vi "PH_SystemInformation.constructor.vi"(0 "name":string, 2 "data in":string, 5 "error in(no error)":errorcluster) -> (14 "i ref out":refnum<vi>, 16 "data out":string, 19 "error out":errorcluster)   [LabVIEW 2014, in "PH_SystemInformation.lvlib"]
doc: "This class is forseen to control black boxes (motion).\n\nThis class is part of the PHELIX device layer.\n\nauthor: Stefan Götte, GSI\n\nLicense Agreement for this software:\n\nCopyright (C)\nGesellschaft für Schwerionenforschung, GSI\nPlanckstr. 1\n64291 Darmstadt\nGermany\n\nContact: D.Beck@gsi.de \n\nThis program is free software; you can redistribute it and/or modify it under the terms of the \nGNU General Public License as published by the Free Software Foundation; either version 2 of \nthe license, or (at your option) any later version.\n\nThis program is distributed in the hope that it will be useful, but WITHOUT ANY WARRANTY; \nwithout even the implied warranty of MERCHANTABILITY or FITNESS FOR A PARTICULAR PURPOSE. See the GNU General License for more details (http://www.gnu.org).\n\nGesellschaft für Schwerionenforschung, GSI\nPlanckstr. 1, 64291 Darmstadt, Germany\nFor all questions and ideas contact: M.Richter@gsi.de, H.Brand@gsi.de or D.Beck@gsi.de.\nLast update: 16-JUN-2004"
uses:
  PH_SystemInformation.lvlib
  CSCore/CSSystem/CSSystemLib/CSSystemLib.lvlib
  PH_Class/PH_Class.lvlib
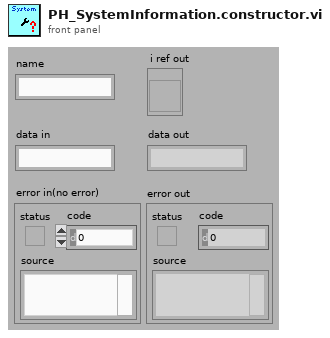
[diagram p1: front panel]
types:
  T1 = enum16{"SetAttribute", "GetAttribute", "CreateAttribute", "DestroyAttribute", "DestroyAllAtributes"}
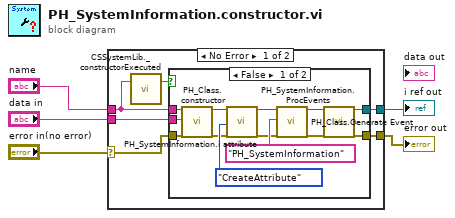
[diagram p0: block diagram]
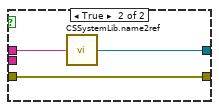
[diagram p2: hidden frame]
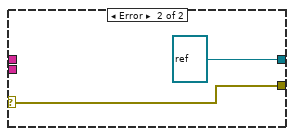
[diagram p3: hidden frame]
diagram:
  n1 = case shown="No Error" "error in(no error)" {
    selector: "error in(no error)" -> [w11 w29]
    tunnel: [w9 refnum<vi> refnum ("i ref out")] -> w5
    tunnel: [w10 w29] -> w4
    tunnel: "name" -> [w8 _]
    tunnel: "data in" -> [w6 _]
    frame No Error {
      n2 = call "CSSystemLib._constructorExecuted.vi"("name"=w8) -> ("constructor executed?"=w7:bool)  [unwired: 18 in]
      n3 = case shown="False" w7 {
        tunnel: w11 -> [w13 w27]
        tunnel: [w23 w27] -> w10
        tunnel: [w22 w25] -> w9
        tunnel: w8 -> [w21 w26]
        tunnel: w6 -> [w12 _]
        frame False {
          n4 = call "PH_Class.constructor.vi"("name"=w21, "data in"=w12, "error in"=w13) -> ("i ref out"=w18:refnum<vi>, "error out"=w19:errorcluster)  [unwired: 14 in, 1 out]
          n5 = call "PH_SystemInformation.i attribute.vi"("VI Refnum"=w18, "Action"=T1."CreateAttribute", "error in (no error)"=w19) -> ("VI Refnum out"=w17:refnum<vi>, "error out"=w16:errorcluster)  [unwired: 14 in, 1 out]
          n6 = call "PH_Class.Generate Event.vi"("i ref in"=w17, "Class"="PH_SystemInformation", "error in (no error)"=w16) -> ("i ref out"=w14:refnum<vi>, "error out"=w15:errorcluster)  [unwired: 15 in]
          n7 = call "PH_SystemInformation.ProcEvents.vi"("i ref in"=w14, "error in (no error)"=w15) -> ("i ref out"=w22:refnum<vi>, "error out"=w23:errorcluster)  [unwired: 16 in]
        }
        frame True {
          n8 = call "CSSystemLib.name2ref.vi"("name"=w26) -> ("obj refnum"=w25:refnum<vi>)
        }
      }
    }
    frame Error {
    }
  }
  "i ref out" <- w5
  "error out" <- w4
